vi "1K pot drainer.vi"() -> ()   [LabVIEW 2021]
uses:
  <userlib>/Nanonis Prog Interface V5/Nanonis Prog Interface.lvlib
panel:
  in  "Milliseconds to wait":i32
  out "Quiet?":bool
  out "Drained?":bool
  out "Current (A)":dbl format="%#_6p"
  in  "Noise threshold (A)":dbl format="%#_6p"
  in  "Equilibrium voltage (V)":dbl=6.8
  in  "Drain voltage (V)":dbl=10.0
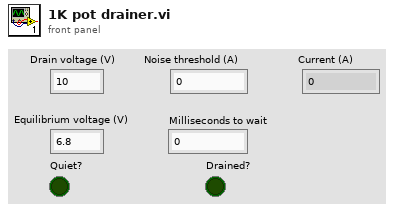
[diagram p1: front panel]
types:
  T1 = enum16{"Set Heater Voltage", "Read Heater Voltage", "Read Heater Current", "Read 1K Pot Temperature", "Read IVC Sorb Temperature", "Read Needle Valve Temperature", "Read Still Pressure", "Read Mixing Chamber Temperature", "Read STM RX Temperature", "Read STM CX Temperature", "Unstall Triton Loop", "Triton Stop", "Triton Stall Status"}
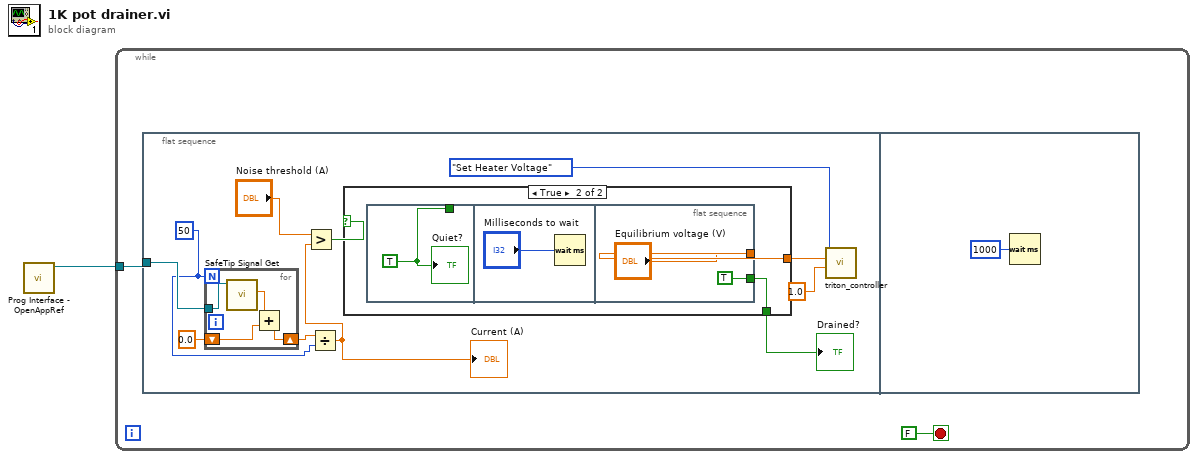
[diagram p0: block diagram]
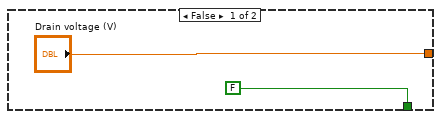
[diagram p2: hidden frame]
diagram:
  n1 = call <userlib>:"Prog Interface - OpenAppRef.vi"() -> ("Application reference"=w1:refnum<vi>)  [unwired: 6 in, 1 out]
  n2 = while {
    tunnel: w1 -> [w2]
    stop <- FALSE stop-if-true
    n3 = flat-sequence {
      tunnel: w2 -> [w14]
      frame #0 {
        w5 = 50
        n4 = for {
          N: w5 -> [_]
          tunnel: w14 -> [w18]
          shift-right: [w17] -> w6
          shift-left: sgl 0.0 ("SafeTip signal value") -> [w15]
          n5 = call <userlib>:"SafeTip Signal Get.vi"("Application ref in"=w18) -> ("SafeTip signal value"=w16:sgl)  [unwired: 8 in, 2 out]
          n6 = Add(x=w16, y=w15) -> (x+y=w17:sgl)
        }
        n7 = Divide(x=w6, y=w5) -> (x/y=w4:sgl)
        "Current (A)" <- w4
        n8 = Greater?(x="Noise threshold (A)", y=w4) -> (0:w12:bool)
        n9 = case shown="True" w12 {
          tunnel: ["Drain voltage (V)" w22] -> w11
          tunnel: [FALSE w21] -> w8
          frame False {
          }
          frame True {
            n10 = flat-sequence {
              tunnel: [w23] -> _
              tunnel: ["Equilibrium voltage (V)"] -> w22
              tunnel: [TRUE] -> w21
              frame #0 {
                w23 = TRUE
                "Quiet?" <- w23
              }
              frame #1 {
                n11 = Wait (ms)(milliseconds to wait="Milliseconds to wait") -> ()  [unwired: 1 out]
              }
              frame #2 {
              }
            }
          }
        }
        "Drained?" <- w8
        n12 = call "triton_controller.vi"("Increment"=1.0, "Numerical Argument"=w11, "Command"=T1."Set Heater Voltage") -> ()  [unwired: 8 in, 1 out]
      }
      frame #1 {
        n13 = Wait (ms)(milliseconds to wait=u32 1000) -> ()  [unwired: 1 out]
      }
    }
  }
